vi "myRIO_BRig_RT_dataExp_Tcycle_Selection.vi"() -> (2 "output_Tcycle_Selection":i32)   [LabVIEW 2014]
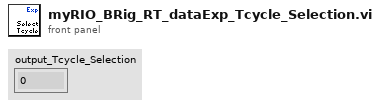
[diagram p1: front panel]
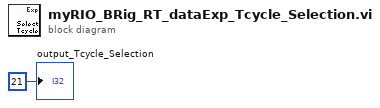
[diagram p0: block diagram]
diagram:
  "output_Tcycle_Selection" <- 21 ("output_iBlock")
